vi "Set Portcullis Piston.vi"(8 "Down":bool, 11 "Up":bool) -> ()   [LabVIEW 2015]
uses:
  <vilib>/Rock Robotics/WPI/Solenoid/WPI_SolenoidValue.ctl
  <vilib>/Rock Robotics/WPI/Solenoid/WPI_SolenoidSetEnum.vi
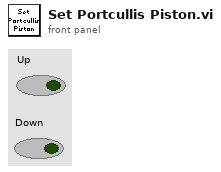
[diagram p1: front panel]
types:
  T1 = typedef "WPI_SolenoidDevRef.ctl" = cluster{"DevStatus":errorcluster, "Pneumatics Control Module":u8, "Forward Solenoid Channel":T2, "Reverse Solenoid Channel":T2}
  T2 = typedef "WPI_SolenoidChannel.ctl" = enum8{"Solenoid 0", "Solenoid 1", "Solenoid 2", "Solenoid 3", "Solenoid 4", "Solenoid 5", "Solenoid 6", "Solenoid 7", "Invalid"}
  T3 = typedef "WPI_SolenoidValue.ctl" = enum16{"Off", "On", "Forward", "Reverse"}
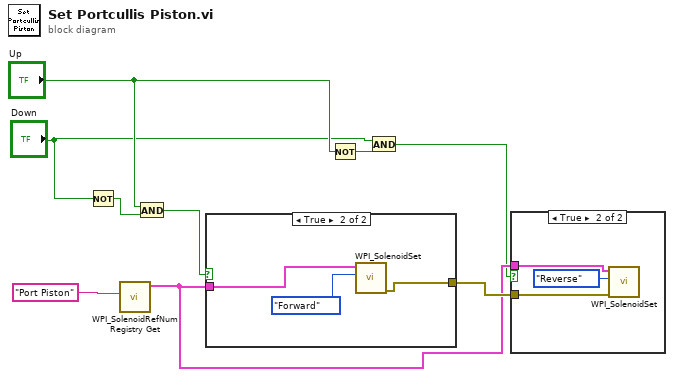
[diagram p0: block diagram]
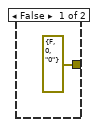
[diagram p3: hidden frame]
diagram:
  n1 = Not(x="Down") -> (.not. x?=w5:bool)
  n2 = call <vilib>:"WPI_SolenoidRefNum Registry Get.vi"("refnum name"="Port Piston") -> ("SolenoidDevRef"=w7:T1)  [unwired: 9 in, 1 out]
  n3 = And(x="Up", y=w5) -> (x .and. y?=w6:bool)
  n4 = case shown="True" w6 {
    tunnel: w7 -> [_ w11]
    tunnel: [errorcluster {"status"=FALSE, "code"=0, "source"="0"} ("error out") w12] -> w9
    frame False {
    }
    frame True {
      n5 = call-poly <vilib>:"WPI_SolenoidSet.vi"("Value"=WPI_SolenoidValue."Forward", "SolenoidDevRef"=w11) -> ("error out"=w12:errorcluster)  [unwired: 8 in, 1 out]
    }
  }
  n6 = Not(x="Up") -> (.not. x?=w3:bool)
  n7 = And(x="Down", y=w3) -> (x .and. y?=w4:bool)
  n8 = case shown="True" w4 {
    tunnel: w7 -> [_ w16]
    tunnel: w9 -> [_ w15]
    frame False {
    }
    frame True {
      n9 = call-poly <vilib>:"WPI_SolenoidSet.vi"("error in (no error)"=w15, "Value"=WPI_SolenoidValue."Reverse", "SolenoidDevRef"=w16) -> ()  [unwired: 7 in, 2 out]
    }
  }
